vi "auxiliar.vi"(1 "posicion":enum16{"5", "4", "3", "2", "1"}(ring), 2 "numPiezas":enum16{"5", "4", "3"}(ring)) -> (0 "posicion":i32)   [LabVIEW 2020]
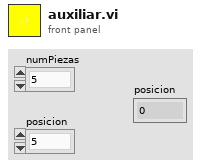
[diagram p1: front panel]
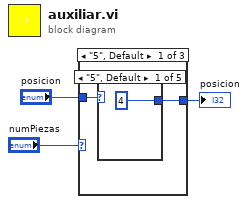
[diagram p0: block diagram]
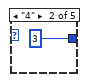
[diagram p2: hidden frame]
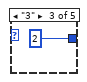
[diagram p3: hidden frame]
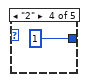
[diagram p4: hidden frame]
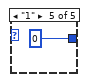
[diagram p5: hidden frame]
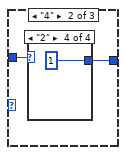
[diagram p6: hidden frame]
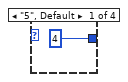
[diagram p7: hidden frame]
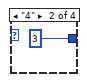
[diagram p8: hidden frame]
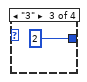
[diagram p9: hidden frame]
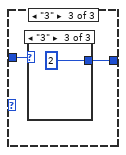
[diagram p10: hidden frame]
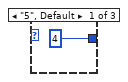
[diagram p11: hidden frame]
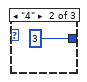
[diagram p12: hidden frame]
diagram:
  n1 = case shown="\"5\", Default" "numPiezas" {
    tunnel: [w5 w11 w17] -> w1
    tunnel: "posicion" -> [w4 w12 w18]
    frame "5", Default {
      n2 = case shown="\"5\", Default" w4 {
        tunnel: [4 3 2 1 0] -> w5
        frame "5", Default {
        }
        frame "4" {
        }
        frame "3" {
        }
        frame "2" {
        }
        frame "1" {
        }
      }
    }
    frame "4" {
      n3 = case shown="\"2\"" w12 {
        tunnel: [4 3 2 1] -> w11
        frame "5", Default {
        }
        frame "4" {
        }
        frame "3" {
        }
        frame "2" {
        }
      }
    }
    frame "3" {
      n4 = case shown="\"3\"" w18 {
        tunnel: [4 3 2] -> w17
        frame "5", Default {
        }
        frame "4" {
        }
        frame "3" {
        }
      }
    }
  }
  "posicion" <- w1
